vi "Trig OP Setup-string convert.vi"(10 "FOR loop index":i32, 11 "Trigger setup element":T1={"Name"="", "Output?"=FALSE, "Output terminal"="/PXI1Slot6/PFI0", "PXI backplane line"="/PXI1Slot6/PXI_Trig0", "Pulse width (us)"=20} {"Pulse width (us)" min=10 max=5000 step=1 format="%.0fµs"}) -> (3 "String":string)   [LabVIEW 2020]
uses:
  Peripherals Control/Triggers/Typedefs/Trigger setup element cluster.ctl
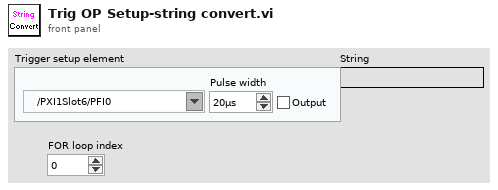
[diagram p1: front panel]
types:
  T1 = typedef "Trigger setup element cluster.ctl" = cluster{"Name":string, "Output?":bool, "Output terminal":tag, "PXI backplane line":tag, "Pulse width (us)":u16}
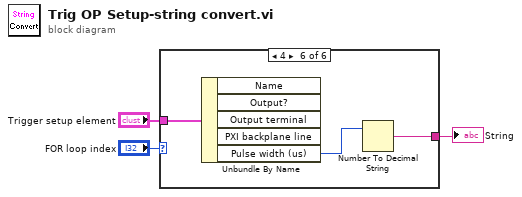
[diagram p0: block diagram]
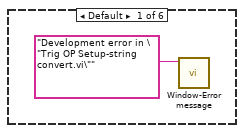
[diagram p2: hidden frame]
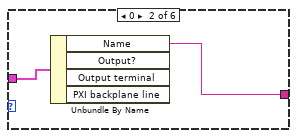
[diagram p3: hidden frame]
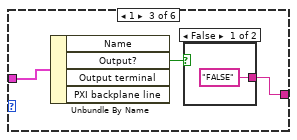
[diagram p4: hidden frame]
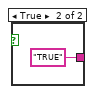
[diagram p5: hidden frame]
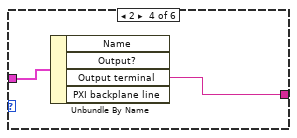
[diagram p6: hidden frame]
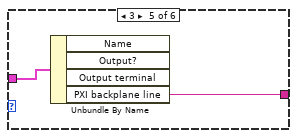
[diagram p7: hidden frame]
diagram:
  n1 = case shown="4" "FOR loop index" {
    tunnel: "Trigger setup element" -> [_ w6 w9 w13 w15 w18]
    tunnel: [_ w5 w8 w12 w14 w16] -> w3
    frame Default {
      n2 = call "Window-Error message.vi"("Message"="Development error in \"Trig OP Setup-string convert.vi\"" ("Error Message")) -> ()  [unwired: 10 in, 1 out]
    }
    frame 0 {
      n3 = Unbundle By Name(w6) -> ("Name"=w5:string)  [unwired: 3 out]
    }
    frame 1 {
      n4 = Unbundle By Name(w9) -> ("Output?"=w7:bool)  [unwired: 3 out]
      n5 = case shown="False" w7 {
        tunnel: ["FALSE" ("Name") "TRUE" ("Name")] -> w8
        frame False {
        }
        frame True {
        }
      }
    }
    frame 2 {
      n6 = Unbundle By Name(w13) -> ("Output terminal"=w12:tag)  [unwired: 3 out]
    }
    frame 3 {
      n7 = Unbundle By Name(w15) -> ("PXI backplane line"=w14:tag)  [unwired: 3 out]
    }
    frame 4 {
      n8 = Unbundle By Name(w18) -> ("Pulse width (us)"=w17:u16)  [unwired: 4 out]
      n9 = Number To Decimal String(number=w17) -> (decimal integer string=w16:string)  [unwired: 1 in]
    }
  }
  "String" <- w3
